vi "Encode String Array.vi"(11 "Strings":string[](array[string])) -> (3 "Encoded String":string)   [LabVIEW 2017]
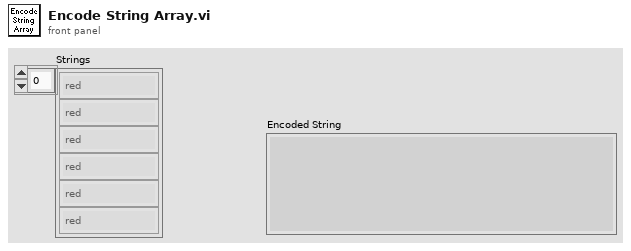
[diagram p1: front panel]
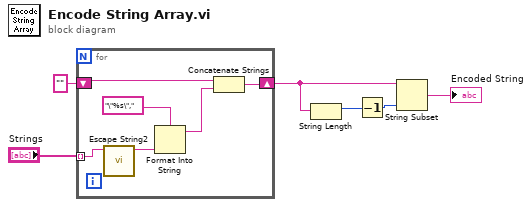
[diagram p0: block diagram]
diagram:
  n1 = for {
    tunnel: "Strings" -> [w8] mode=indexing
    shift-right: [w9] -> w5
    shift-left: "" -> [w10]
    n2 = call <vilib>:"Escape String2.vi"("input"=w8) -> ("output"=w7:string)  [unwired: 10 in]
    n3 = Format Into String(format string="\"%s\",", w7) -> (resulting string=w11:string)  [unwired: 2 in, 1 out]
    n4 = Concatenate Strings(w10, w11) -> (w9:string)
  }
  n5 = String Length(string=w5) -> (length=w3:i32)
  n6 = Decrement(x=w3) -> (x-1=w4:i32)
  n7 = String Subset(string=w5, length (rest)=w4) -> (substring=→"Encoded String":string)  [unwired: 1 in]
